vi "AE - Bluetooth Reorder.vi"(8 "error in (no error)":errorcluster, 10 "No. of Wiimotes Paired":i32, 11 "Reorder Array":i32[](array[numeric])) -> (0 "error out":errorcluster)   [LabVIEW 2010]
uses:
  AE Cores/AE - Bluetooth Enum.ctl
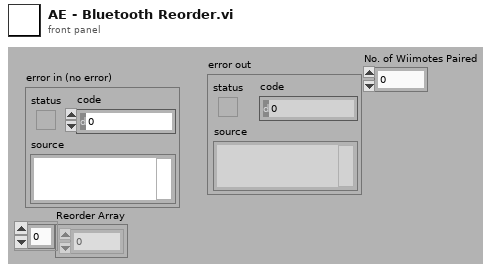
[diagram p1: front panel]
types:
  T1 = typedef "AE - Bluetooth Enum.ctl" = enum16{"Initialise", "Pair All Wiimotes", "Connect All Wiimotes", "Set Rumble", "Set LED", "Get Button + Acc Data", "Get IR Data", "Get Battery", "Get Wiimote Reference", "Reorder Wiimotes", "devReport"}
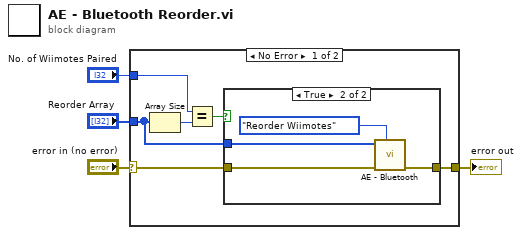
[diagram p0: block diagram]
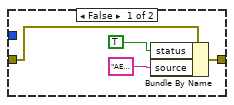
[diagram p2: hidden frame]
diagram:
  n1 = case shown="No Error" "error in (no error)" {
    selector: "error in (no error)" -> [w10 w19]
    tunnel: [w9 w19] -> w3
    tunnel: "Reorder Array" -> [w8 _]
    tunnel: "No. of Wiimotes Paired" -> [w6 _]
    frame No Error {
      n2 = Array Size(array=w8) -> (size(s)=w7:i32)
      n3 = Equal?(x=w6, y=w7) -> (x = y?=w5:bool)
      n4 = case shown="True" w5 {
        tunnel: w10 -> [w14 w17]
        tunnel: [w13 w16] -> w9
        tunnel: w8 -> [_ w15]
        frame False {
          n5 = Bundle By Name(cluster=w14, "status"=TRUE, "source"="AE - Bluetooth Reorder.vi : Reorder Array incorrect size or Null") -> (w13:errorcluster)
        }
        frame True {
          n6 = call "AE - Bluetooth.vi"("Enum"=AE_-_Bluetooth_Enum."Reorder Wiimotes", "error in (no error)"=w17, "Variant In"=w15) -> ("error out"=w16:errorcluster)  [unwired: 6 in, 2 out]
        }
      }
    }
    frame Error {
    }
  }
  "error out" <- w3
